vi "Unit Vector.vi"(10 "Position 2":refnum<class "Vector 2D.lvclass">, 11 "Position 1":refnum<class "Vector 2D.lvclass">) -> (3 "Unit Vector In Direction":refnum<class "Vector 2D.lvclass">)   [LabVIEW 2021, in "Vector 2D.lvclass"]
uses:
  Vector 2D.lvclass
  Vector 2D.lvclass/Vector 2D.ctl
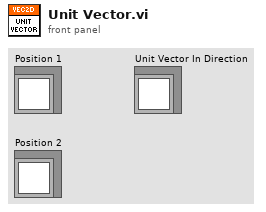
[diagram p1: front panel]
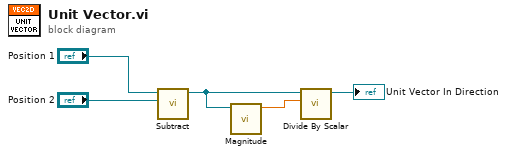
[diagram p0: block diagram]
diagram:
  n1 = call "Subtract.vi"("B"="Position 2", "A"="Position 1") -> ("A-B"=w3:refnum<class "Vector 2D.lvclass">)  [unwired: 9 in]
  n2 = call "Magnitude.vi"("A"=w3) -> ("Magnitude"=w1:sgl)  [unwired: 10 in]
  n3 = call "Divide By Scalar.vi"("x"=w1, "A"=w3) -> ("Ax"=→"Unit Vector In Direction":refnum<class "Vector 2D.lvclass">)  [unwired: 9 in]
